vi "R-T Data Input [Array Control].vi"() -> ()   [LabVIEW 2017]
panel:
  in  "R-T Data":cluster{"T [Celsius]":dbl[], "R [kiohm]":dbl[]}={"T [Celsius]"=[-50.0, -45.0, -40.0, -35.0, -30.0], "R [kiohm]"=[670.1, 471.7, 336.5, 242.6, 177.0]}
  out "XY Graph":cluster{"T [Celsius]":dbl[], "R [kiohm]":dbl[]}(graph)
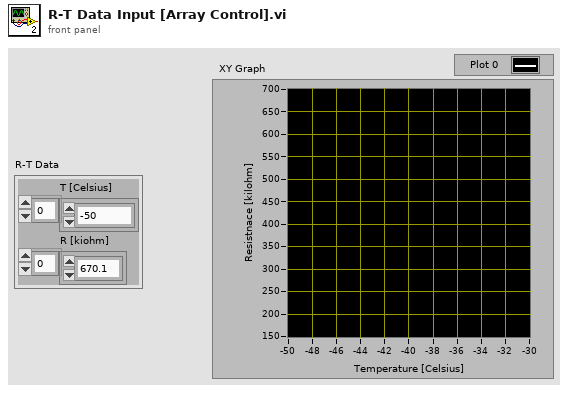
[diagram p1: front panel]
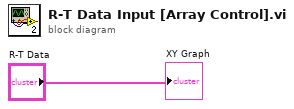
[diagram p0: block diagram]
diagram:
  "XY Graph" <- "R-T Data"
